vi "SendSetReconnectInterval.vi"(8 "error in (no error)":errorcluster, 10 "reconnect interval":dbl, 11 "Qbus in":refnum<class "Qbus.lvclass">) -> (0 "error out":errorcluster, 3 "Qbus out":refnum<class "Qbus.lvclass">)   [LabVIEW 2017, in "ServerComm.lvlib"]
doc: "Sets the amount of time, in seconds, to wait between a failed attempt to connect to NI InsightCM Server and attempts to reconnect."
uses:
  <vilib>/addons/InsightCM/Devices/Shared/Common/ServerComm/ServerComm.lvlib
  <vilib>/addons/Qbus/Qbus.lvclass
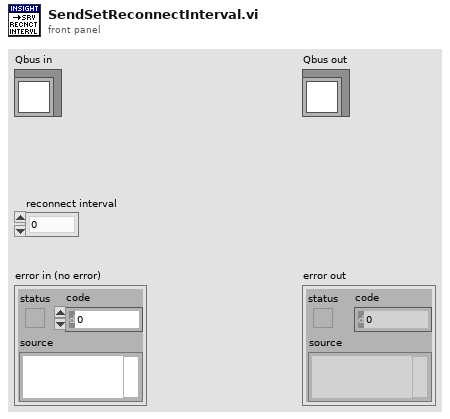
[diagram p1: front panel]
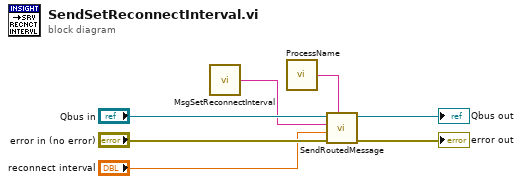
[diagram p0: block diagram]
diagram:
  n1 = call <vilib>:"MsgSetReconnectInterval.vi"() -> ("message name"=w1:string)  [unwired: 5 in]
  n2 = call <vilib>:"ProcessName.vi"() -> ("process name"=w4:string)  [unwired: 5 in]
  n3 = call <vilib>:"SendRoutedMessage.vi"("listener process"=w4, "error in (no error)"="error in (no error)", "message value"="reconnect interval", "message name"=w1, "Qbus in"="Qbus in") -> ("error in (no error)"=→"error out":errorcluster, "Qbus out"=→"Qbus out":refnum<class "Qbus.lvclass">)  [unwired: 5 in]
